vi "AutoIndexing.vi"() -> ()   [LabVIEW 2019]
panel:
  out "element":dbl
  in  "Array":dbl[](array[numeric])
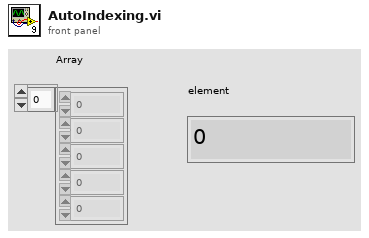
[diagram p1: front panel]
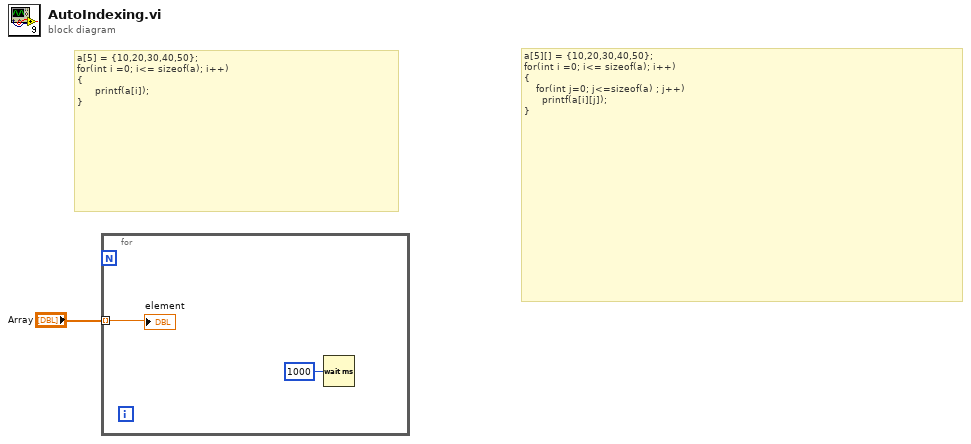
[diagram p0: block diagram]
diagram:
  # "a[5][] = {10,20,30,40,50};\nfor(int i =0; i<= sizeof(a); i++)\n{\n    for(int j=0; j<=sizeof(a) ; j++)\n      printf(a[i][j]);\n}"
  # "a[5] = {10,20,30,40,50};\nfor(int i =0; i<= sizeof(a); i++)\n{\n      printf(a[i]);\n}"
  n1 = for {
    tunnel: "Array" -> [w2] mode=indexing
    n2 = Wait (ms)(milliseconds to wait=u32 1000) -> ()  [unwired: 1 out]
    "element" <- w2
  }
